vi "Sample Math & Signal Processing Algorithm.vi"(9 "signal size":i32=10, 10 "matrix size":i32=10, 11 "iteration":i32=10) -> (2 "max difference":dbl, 3 "Time Per Iteration":u32[](array[numeric]))   [LabVIEW 2023]
doc: "Implements a sample algorithm to be executed within the RT Analysis Workspace."
uses:
  <vilib>/Analysis/7linalg.llb/Real Transpose Matrix.vi
  <vilib>/Analysis/baseanly.llb/Real A x B.vi
  <vilib>/Analysis/4window.llb/Modified Bartlett-Hanning Window (DBL).vi
  Instance           1 49Saved   Sample Math & Signal Processing Algorithm .vi
  <vilib>/Analysis/7linalg.llb/Real Eigenvalues and Vectors.vi
  <vilib>/Analysis/7linalg.llb/Real SVD Decomposition.vi
  Instance           2 49Saved   Sample Math & Signal Processing Algorithm .vi
  <vilib>/Analysis/NI_AALPro.lvlib
  <vilib>/Analysis/NI_AALBase.lvlib
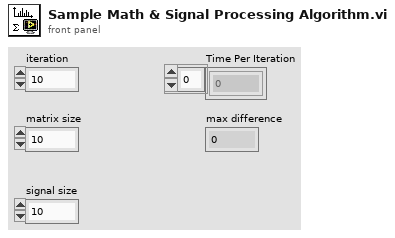
[diagram p1: front panel]
types:
  T1 = typedef "NI_Matrix.lvlib/RealMatrix.ctl" = dbl[][]
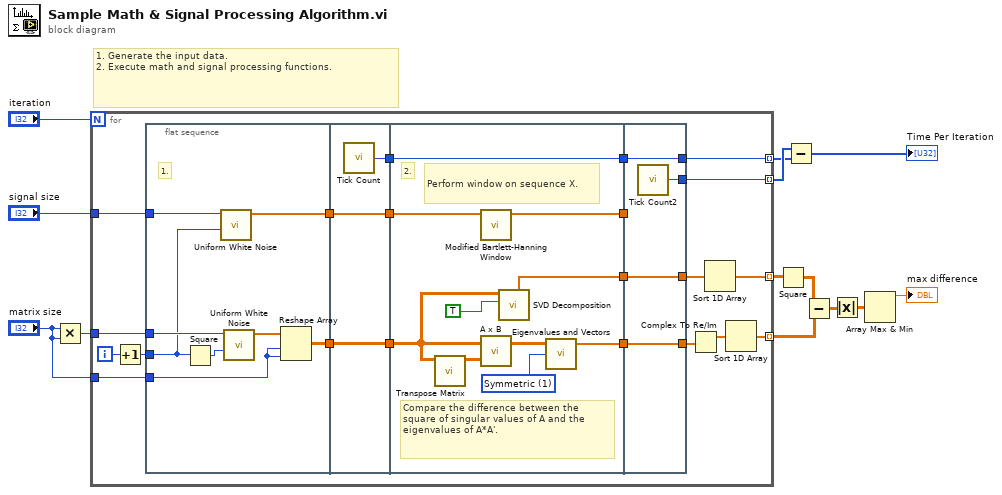
[diagram p0: block diagram]
diagram:
  # "1. Generate the input data.\n2. Execute math and signal processing functions."
  n1 = Multiply(x="matrix size", y="matrix size") -> (x*y=w9:i32)
  n2 = for {
    N: "iteration" -> [_]
    tunnel: [w34] -> w12 mode=indexing
    tunnel: "signal size" -> [w33]
    tunnel: w9 -> [w30]
    tunnel: "matrix size" -> [w29]
    tunnel: [w21] -> w7 mode=indexing
    tunnel: [w17] -> w5 mode=indexing
    tunnel: [w16] -> w1 mode=indexing
    i -> [w32]
    n3 = Increment(x=w32) -> (x+1=w31:i32)
    n4 = flat-sequence {
      tunnel: w29 -> [w38]
      tunnel: w30 -> [w39]
      tunnel: w31 -> [w35]
      tunnel: w33 -> [w40]
      tunnel: [w37] -> w27
      tunnel: [w36] -> w25
      tunnel: w27 -> [w45]
      tunnel: [w45] -> w26
      tunnel: w25 -> [w44]
      tunnel: [w44] -> w24
      tunnel: [w43] -> w14
      tunnel: [w55] -> w28
      tunnel: w26 -> [w54]
      tunnel: w24 -> [w51]
      tunnel: [w48] -> w23
      tunnel: [w47] -> w22
      tunnel: [w46] -> w15
      tunnel: w14 -> [w46]
      tunnel: [w59] -> w34
      tunnel: w28 -> [_]
      tunnel: [w58] -> w19
      tunnel: w23 -> [w58]
      tunnel: [w57] -> w20
      tunnel: w22 -> [w57]
      tunnel: [w56] -> w16
      tunnel: w15 -> [w56]
      frame #0 {
        # "1."
        n5 = Square(x=w35) -> (x^2=w42:i32)
        n6 = call <vilib>:"Uniform White Noise.vi"("seed"=w35, "samples"=w40) -> ("uniform white noise"=w37:dbl[])  [unwired: 8 in, 1 out]
        n7 = call <vilib>:"Uniform White Noise.vi"("seed"=w42, "samples"=w39) -> ("uniform white noise"=w41:dbl[])  [unwired: 8 in, 1 out]
        n8 = Reshape Array(w41, w38, w38) -> (w36:dbl[][])
      }
      frame #1 {
        n9 = call "Tick Count"() -> ("Tick Count(uSec)"=w43:u32)
      }
      frame #2 {
        w49 = 1 items=["General", "Symmetric"] ("matrix type")
        # "Compare the difference between the square of singular values of A and the eigenvalues of A*A'."
        # "Perform window on sequence X."
        # "2."
        n10 = call-poly <vilib>:"Transpose Matrix.vi"("Input Matrix"=w51) -> ("Matrix Transpose"=w53:T1)  [unwired: 9 in, 1 out]
        n11 = call-poly <vilib>:"Modified Bartlett-Hanning Window.vi"("X"=w54) -> ("Windowed X"=w55:dbl[])  [unwired: 9 in, 1 out]
        n12 = call-poly <vilib>:"A x B.vi"("B"=w53, "A"=w51) -> ("A x B"=w50:T1)  [unwired: 1 out]
        n13 = call-poly <vilib>:"SVD Decomposition.vi"("singular values only?"=TRUE, "A"=w51) -> ("Vector S"=w47:dbl[])  [unwired: 5 in, 4 out]
        n14 = call-poly <vilib>:"Eigenvalues and Vectors.vi"("matrix type"=w49, "Input Matrix"=w50) -> ("Eigenvalues"=w48:cdb[])  [unwired: 1 in, 2 out]
      }
      frame #3 {
        n15 = call "Tick Count2"() -> ("Tick Count(uSec)"=w59:u32)
      }
    }
    n16 = Complex To Re/Im(x + iy=w19) -> (x=w18:dbl[])  [unwired: 1 out]
    n17 = Sort 1D Array(array=w20) -> (sorted array=w21:dbl[])
    n18 = Sort 1D Array(array=w18) -> (sorted array=w17:dbl[])
  }
  n19 = Square(x=w7) -> (x^2=w6:dbl[][])
  n20 = Subtract(x=w12, y=w1) -> (x-y=→"Time Per Iteration":u32[])
  n21 = Subtract(x=w6, y=w5) -> (x-y=w4:dbl[][])
  n22 = Absolute Value(x=w4) -> (abs(x)=w3:dbl[][])
  n23 = Array Max & Min(array=w3) -> (max value=→"max difference":dbl)  [unwired: 3 out]
